vi "dll_path.vi"() -> (2 "dll":path=path "C:/code/LabVIEW-MIDI-XPLAT/dist/TomMIDIllan_64.dll")   [LabVIEW 2020, in "MIDIllan.lvlib"]
uses:
  MIDIllan.lvlib
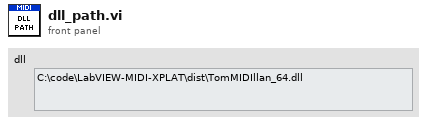
[diagram p1: front panel]
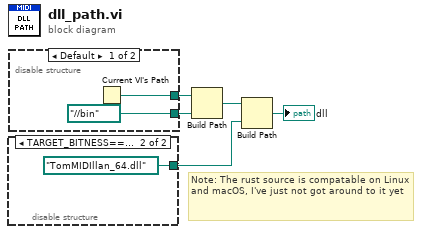
[diagram p0: block diagram]
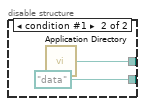
[diagram p2: hidden frame]
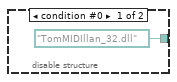
[diagram p3: hidden frame]
diagram:
  # "Note: The rust source is compatable on Linux and macOS, I've just not got around to it yet"
  n1 = disable-structure shown="TARGET_BITNESS==64" {
    disable-tunnel: [path "TomMIDIllan_32.dll" ("dll") path "TomMIDIllan_64.dll" ("dll")] -> w4
    frame condition #0 {
    }
    frame condition #1 (active) {
    }
  }
  n2 = disable-structure shown="Default" {
    disable-tunnel: [path "../../bin" ("name or relative path") path "data" ("name or relative path")] -> w3
    disable-tunnel: [w9 w10] -> w1
    frame condition #0 (active) {
      n3 = Current VI's Path() -> (path=w9:path)
    }
    frame condition #1 {
      n4 = call <vilib>:"Application Directory.vi"() -> ("Application Directory"=w10:path)
    }
  }
  n5 = Build Path(base path=w1, name or relative path=w3) -> (appended path=w2:path)
  n6 = Build Path(base path=w2, name or relative path=w4) -> (appended path=→"dll":path)
